vi "dataAcquiqition.vi"(0 "Background image handle":u32, 1 "Image Handle":u32, 2 "Camera Handle":u32, 3 "Error IN":errorcluster caption="entrée d'erreur (pas d'erreur)", 4 "Strip number":u32) -> (7 "Camera handle":i32, 8 "Image Handle":u32, 10 "Error OUT":errorcluster caption="sortie d'erreur")   [LabVIEW 2020]
panel:
  out "Nb abscissa pixels":i32
  in  "SITKFULLDISPLAYLib.SITKFullDisplay":refnum<k7>(container)
  in  "Use background":bool
  out "Graphe":u16[][](graph)
  in  "Stop acquisiton":bool
  # "Strips spectral"
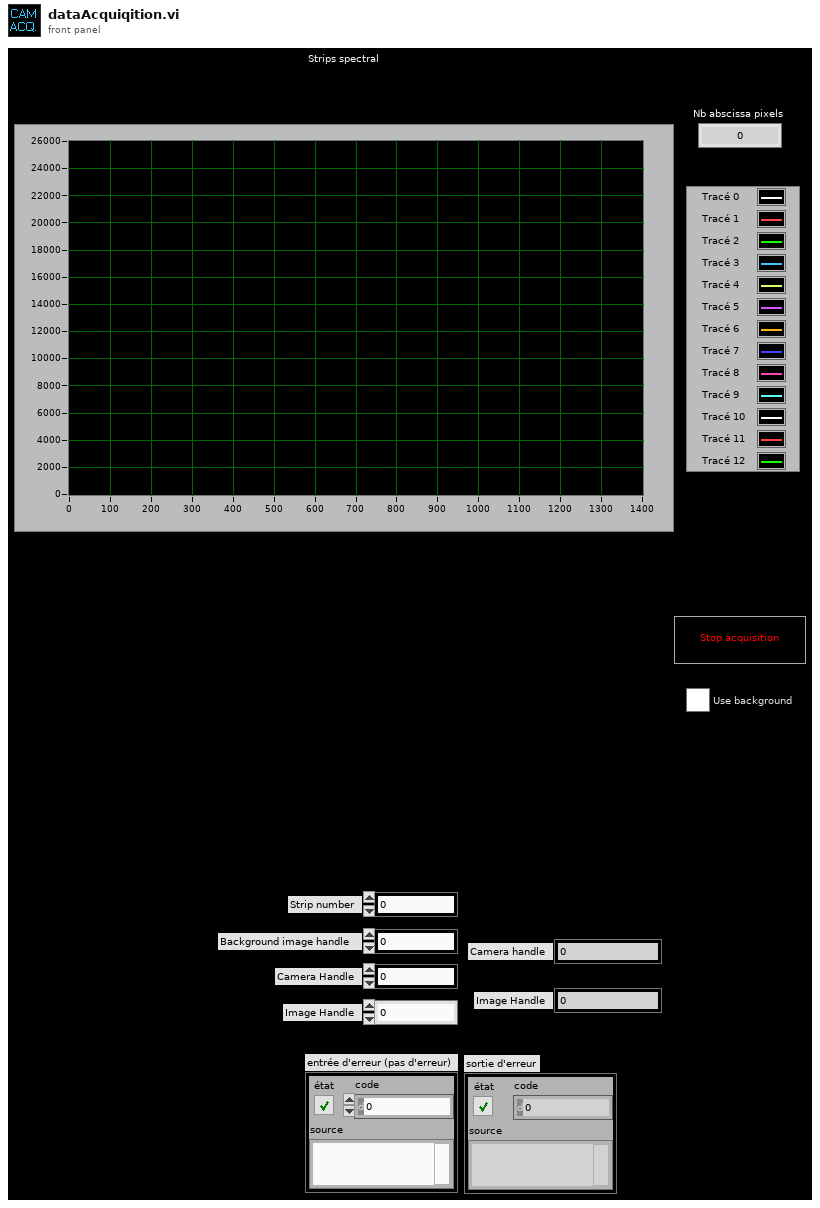
[diagram p1: front panel]
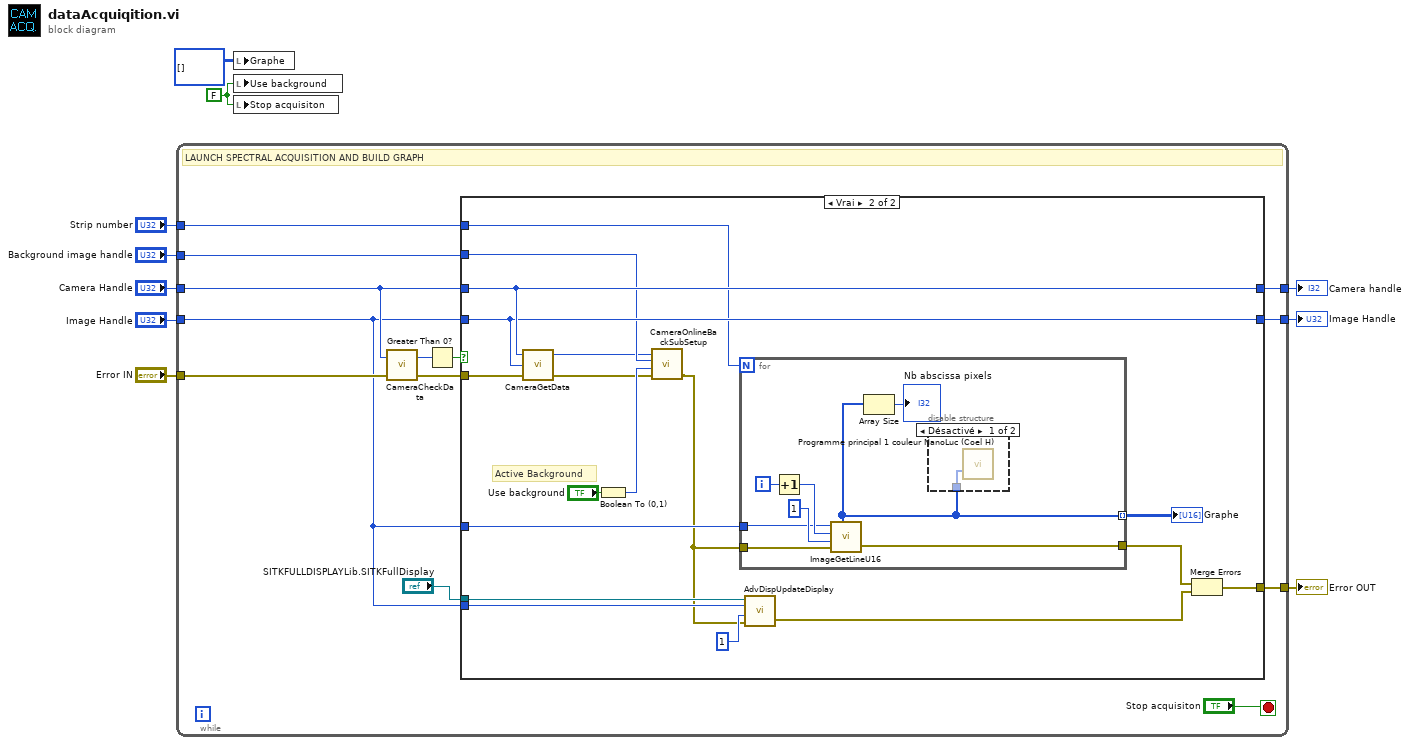
[diagram p0: block diagram]
diagram:
  w5 = FALSE ("Stop acquisiton")
  n1 = while {
    tunnel: "Error IN" -> [w15]
    tunnel: "Image Handle" -> [w11]
    tunnel: "Camera Handle" -> [w13]
    tunnel: [w21] -> w8
    tunnel: [w20] -> w10
    tunnel: [w19] -> w9
    tunnel: "Background image handle" -> [w14]
    tunnel: "Strip number" -> [w12]
    stop <- "Stop acquisiton" stop-if-true
    # "LAUNCH SPECTRAL ACQUISITION AND BUILD GRAPH"
    n2 = call <userlib>:"CameraCheckData.vi"("Camera Handle"=w13, "error in"=w15) -> ("Number Of Frames Available"=w16:i32, "error out"=w23:errorcluster)  [unwired: 1 out]
    n3 = Greater Than 0?(x=w16) -> (x > 0?=w22:bool)
    n4 = case shown="Vrai" w22 {
      tunnel: w23 -> [w26 w44]
      tunnel: w11 -> [w24 w37]
      tunnel: w13 -> [w25 w38]
      tunnel: [w26 w28] -> w21
      tunnel: [w25 w38] -> w20
      tunnel: [w24 w37] -> w19
      tunnel: "SITKFULLDISPLAYLib.SITKFullDisplay" -> [_ w43]
      tunnel: w14 -> [_ w36]
      tunnel: w12 -> [_ w27]
      tunnel: w11 -> [_ w34]
      tunnel: w11 -> [_ w32]
      frame False {
      }
      frame True {
        # "Active Background"
        n5 = call <userlib>:"CameraGetData.vi"("error in"=w44, "Image/Data Handle"=w37, "Camera Handle"=w38) -> ("error out"=w39:errorcluster, "Camera Handle"=w33:u32)  [unwired: 1 out]
        n6 = Boolean To (0,1)(Boolean="Use background") -> (0, 1=w41:i16)
        n7 = call <userlib>:"CameraOnlineBackSubSetup.vi"("error in"=w39, "Background Flag"=w41, "Background Image Handle"=w36, "Camera Handle"=w33) -> ("error out"=w31:errorcluster)  [unwired: 2 out]
        n8 = for {
          N: w27 -> [_]
          tunnel: w32 -> [w49]
          tunnel: [w46] -> w35 mode=indexing
          tunnel: w31 -> [w48]
          tunnel: [w47] -> w30
          i -> [w52]
          n9 = Increment(x=w52) -> (x+1=w51:i32)
          n10 = call <userlib>:"ImageGetLineU16.vi"("Data Handle"=w49, "Y Position"=w51, "Z Position"=u32 1, "error in"=w48) -> ("Array u16"=w46:u16[], "error out"=w47:errorcluster)  [unwired: 1 out]
          n11 = Array Size(array=w46) -> (size(s)=→"Nb abscissa pixels":i32)
          n12 = disable-structure shown="Désactivé" {
            disable-tunnel: w46 -> [w53 _]
            frame Disabled {
              n13 = call "Programme principal 1 couleur NanoLuc (Coel H).vi"("Y"=w53) -> ()  [unwired: 13 in, 2 out]
            }
            frame Enabled {
            }
          }
        }
        "Graphe" <- w35
        n14 = call <userlib>:"AdvDispUpdateDisplay.vi"("error in (no error)"=w31, "Frame Number To Display"=u32 1, "Image Handle"=w34, "SITKFULLDISPLAYLib.SITKFullDisplay"=w43) -> ("error out"=w29:errorcluster)  [unwired: 1 out]
        n15 = Merge Errors(w30, w29) -> (w28:errorcluster)
      }
    }
  }
  "Camera handle" <- w10
  "Image Handle" <- w9
  "Error OUT" <- w8
  n16 = local write "Graphe"(i32[][] [] ("Graphe")) -> ()
  n17 = local write "Use background"(w5) -> ()
  n18 = local write "Stop acquisiton"(w5) -> ()
